vi "LVClass_Pupil Apply Shut of Boundaries.vi"(0 "Pupil in":refnum<class "Pupil.lvclass">, 7 "ShutOfBoundaries":u32, 11 "error in (no error)":errorcluster) -> (4 "Pupil out":refnum<class "Pupil.lvclass">, 15 "error out":errorcluster)   [LabVIEW 2020, in "Pupil.lvclass"]
uses:
  Pupil.lvclass
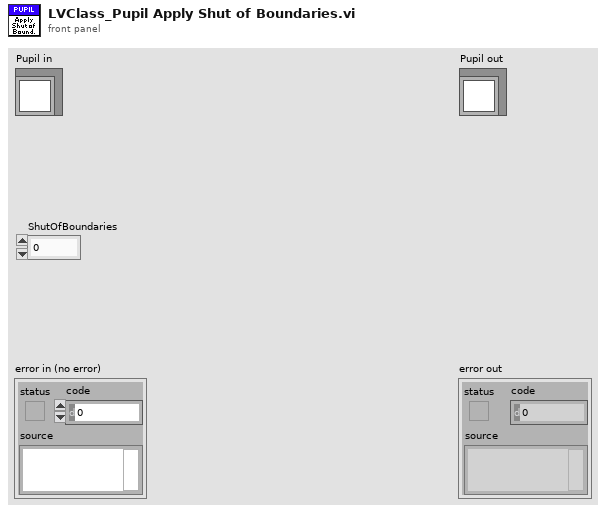
[diagram p1: front panel]
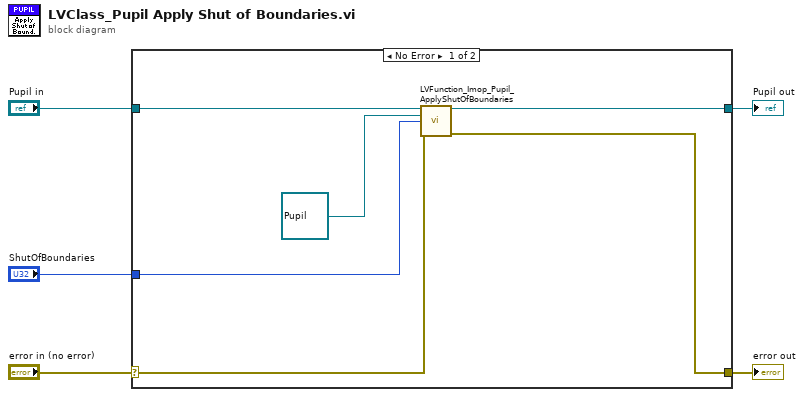
[diagram p0: block diagram]
diagram:
  n1 = case shown="No Error" "error in (no error)" {
    selector: "error in (no error)" -> [w9 w13]
    tunnel: [w7 w13] -> w4
    tunnel: [w8 w12] -> w2
    tunnel: "Pupil in" -> [w10 w12]
    tunnel: "ShutOfBoundaries" -> [w11 _]
    frame No Error {
      n2 = call "LVFunction_Imop_Pupil_ApplyShutOfBoundaries.vi"("Pupil in"=w10, "Pupil OUT"=refnum<class "Pupil.lvclass"> refnum, "ShutOfBoundaries"=w11, "error in (no error)"=w9) -> ("Pupil out"=w8:refnum<class "Pupil.lvclass">, "error out"=w7:errorcluster)  [unwired: 9 in, 1 out]
    }
    frame Error {
    }
  }
  "error out" <- w4
  "Pupil out" <- w2
